vi "AcquisitionDone.vi"(8 "error in (no error)":errorcluster, 10 "Acq Done Data":T1, 11 "CommToUI in":refnum<class "CommToUI.lvclass">) -> (0 "error out":errorcluster, 3 "CommToUI out":refnum<class "CommToUI.lvclass">)   [LabVIEW 2023, in "ControllerComm.lvlib" / "CommToUI.lvclass"]
uses:
  Controller Comm/CommToUI.lvclass
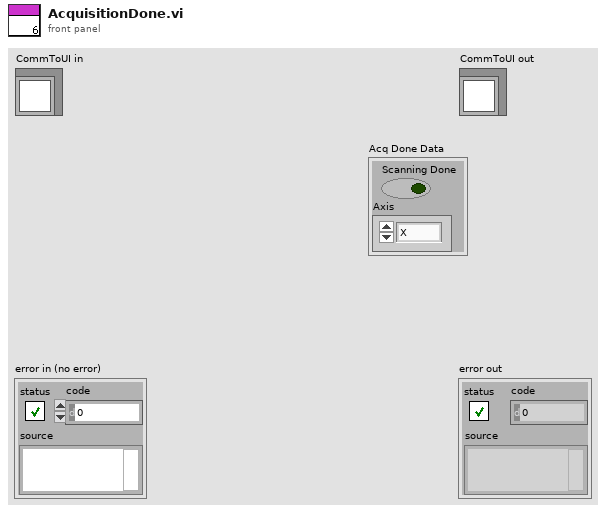
[diagram p1: front panel]
types:
  T1 = cluster{"Scanning Done":bool, "Axis":enum16{"X", "Y", "Z", "HOM"}}
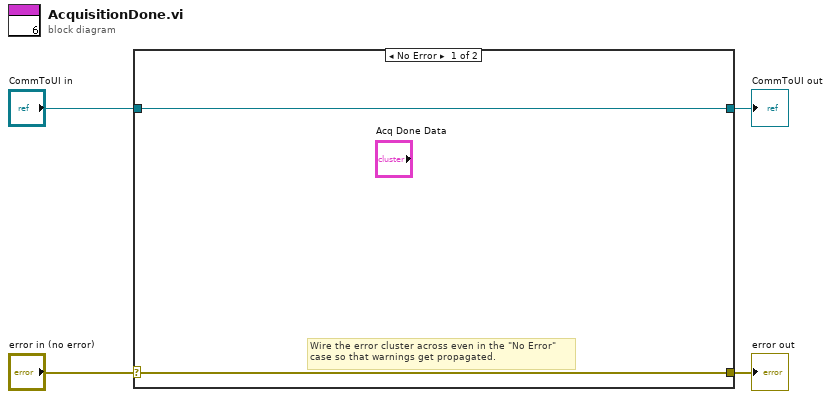
[diagram p0: block diagram]
diagram:
  n1 = case shown="No Error" "error in (no error)" {
    selector: "error in (no error)" -> [w5 w8]
    tunnel: [w5 w8] -> w3
    tunnel: [w6 w7] -> w1
    tunnel: "CommToUI in" -> [w6 w7]
    frame No Error {
      # "Wire the error cluster across even in the \"No Error\"\ncase so that warnings get propagated."
    }
    frame Error {
    }
  }
  "error out" <- w3
  "CommToUI out" <- w1
